vi "Generate Simulated Data.vi"(8 "error in (no error)":errorcluster) -> (0 "error out":errorcluster, 2 "Graph Data":waveform(dbl)[](array[waveform]))   [LabVIEW 2018, in "DAQ Device.lvlib"]
doc: "Generates sample waveforms according to the signal type in the HW Config input.\n_____\nBased on Delacor QMH Project Template 4.2.0.62."
uses:
  DAQ Device.lvlib
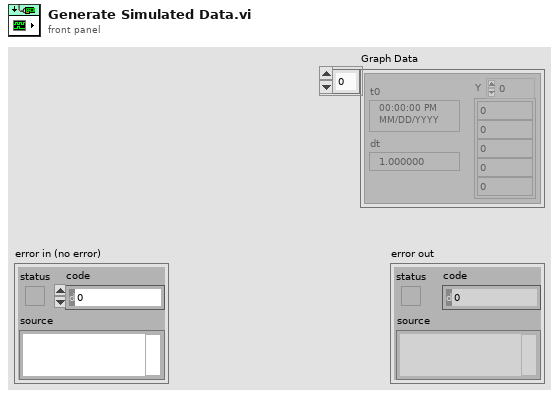
[diagram p1: front panel]
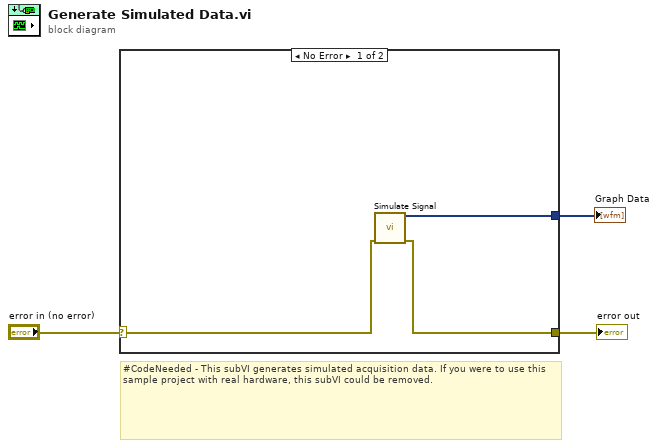
[diagram p0: block diagram]
diagram:
  # "#CodeNeeded - This subVI generates simulated acquisition data. If you were to use this sample project with real hardware, this subVI could be removed."
  n1 = case shown="No Error" "error in (no error)" {
    selector: "error in (no error)" -> [w5 w7]
    tunnel: [w4 w7] -> w2
    tunnel: [w6 _] -> w1
    frame No Error {
      n2 = call "Simulate Signal"("error in (no error)"=w5) -> ("Sine"=w6:dynamicdata, "error out"=w4:errorcluster)  [unwired: 13 in]
    }
    frame Error {
    }
  }
  "error out" <- w2
  "Graph Data" <- w1
